vi "CaseVI.vi"() -> ()   [LabVIEW 2019]
uses:
  myEnum.ctl
  myLibrary.lvlib
panel:
  in  "String":string
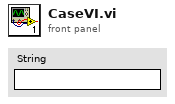
[diagram p1: front panel]
types:
  T1 = typedef "myLibrary.lvlib/myEnum.ctl" = enum16{"Item1", "Item 2", "Item 3"}
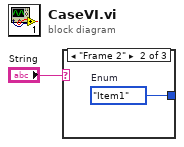
[diagram p0: block diagram]
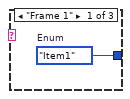
[diagram p2: hidden frame]
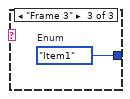
[diagram p3: hidden frame]
diagram:
  n1 = case shown="\"Frame 2\"" "String" {
    tunnel: [w2 w3 w4] -> _
    frame "Frame 1" {
      w2 = myEnum."Item1"  # Enum
    }
    frame "Frame 2" {
      w3 = myEnum."Item1"  # Enum
    }
    frame "Frame 3" {
      w4 = myEnum."Item1"  # Enum
    }
  }
